vi "sub_ofdm_subcarrier_partitioner.vi"(8 "pilot carrier":i32, 9 "message carrier":i32, 10 "FFT size":i32, 11 "received symbol":cdb[](array[numeric])) -> (0 "pilot subcarriers":cdb[](array[numeric]), 3 "message subcarriers":cdb[](array[numeric]))   [LabVIEW 2014]
panel:
  out "message size":i32
  out "Pilot size":i32
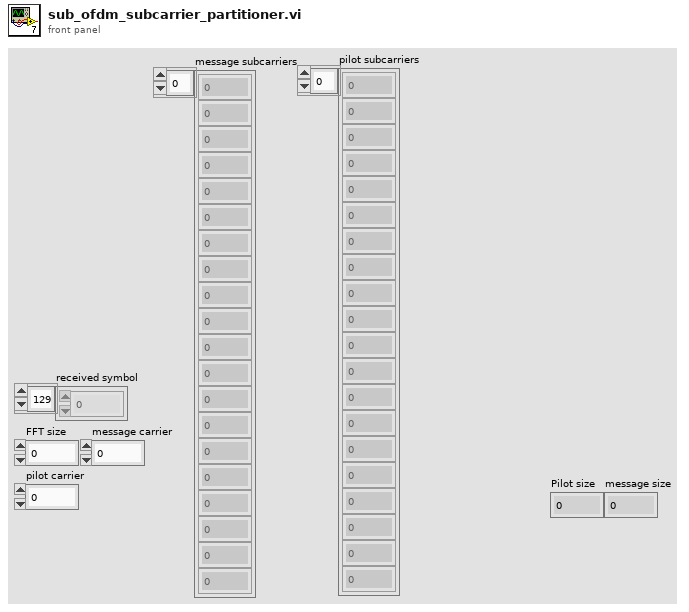
[diagram p1: front panel]
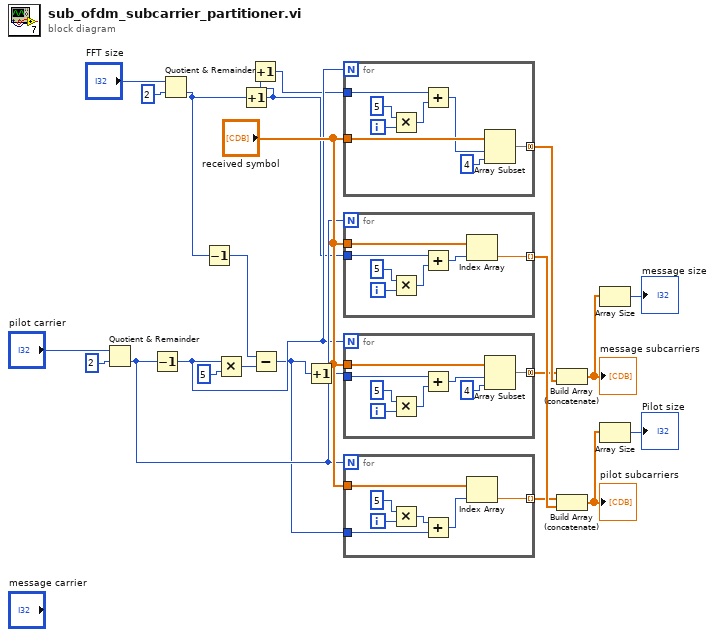
[diagram p0: block diagram]
diagram:
  n1 = Quotient & Remainder(x="pilot carrier", y=2) -> (floor(x/y)=w8:i32)  [unwired: 1 out]
  n2 = Decrement(x=w8) -> (x-1=w7:i32)
  n3 = Quotient & Remainder(x="FFT size", y=2) -> (floor(x/y)=w5:i32)  [unwired: 1 out]
  n4 = Decrement(x=w5) -> (x-1=w6:i32)
  n5 = Multiply(x=w7, y=5) -> (x*y=w17:i32)
  n6 = Increment(x=w5) -> (x+1=w3:i32)
  n7 = Increment(x=w3) -> (x+1=w4:i32)
  n8 = Subtract(x=w6, y=w17) -> (x-y=w1:i32)
  n9 = Increment(x=w1) -> (x+1=w2:i32)
  n10 = for {
    N: w7 -> [_]
    tunnel: w4 -> [w29]
    tunnel: "received symbol" -> [w31]
    tunnel: [w28] -> w15 mode=concatenating
    i -> [w26]
    n11 = Multiply(x=5, y=w26) -> (x*y=w27:i32)
    n12 = Add(x=w29, y=w27) -> (x+y=w30:i32)
    n13 = Array Subset(array=w31, index=w30, length=4) -> (w28:cdb[])
  }
  n14 = for {
    N: w8 -> [_]
    tunnel: w3 -> [w37]
    tunnel: "received symbol" -> [w36]
    tunnel: [w32] -> w19 mode=indexing
    i -> [w35]
    n15 = Multiply(x=5, y=w35) -> (x*y=w34:i32)
    n16 = Add(x=w37, y=w34) -> (x+y=w38:i32)
    n17 = Index Array(array=w36, index=w38) -> (element=w32:cdb)
  }
  n18 = for {
    N: w7 -> [_]
    tunnel: "received symbol" -> [w44]
    tunnel: w2 -> [w41]
    tunnel: [w39] -> w13 mode=concatenating
    i -> [w45]
    n19 = Multiply(x=5, y=w45) -> (x*y=w42:i32)
    n20 = Add(x=w41, y=w42) -> (x+y=w43:i32)
    n21 = Array Subset(array=w44, index=w43, length=4) -> (w39:cdb[])
  }
  n22 = for {
    N: w8 -> [_]
    tunnel: "received symbol" -> [w53]
    tunnel: w1 -> [w51]
    tunnel: [w50] -> w16 mode=indexing
    i -> [w49]
    n23 = Multiply(x=5, y=w49) -> (x*y=w48:i32)
    n24 = Add(x=w48, y=w51) -> (x+y=w52:i32)
    n25 = Index Array(array=w53, index=w52) -> (element=w50:cdb)
  }
  n26 = Build Array (concatenate)(w13, w15) -> (w10:cdb[])
  "message subcarriers" <- w10
  n27 = Build Array (concatenate)(w16, w19) -> (w12:cdb[])
  "pilot subcarriers" <- w12
  n28 = Array Size(array=w10) -> (size(s)=→"message size":i32)
  n29 = Array Size(array=w12) -> (size(s)=→"Pilot size":i32)
